vi "Configure Valve Output.vi"(8 "error in (no error)":errorcluster, 9 "valve output, %":sgl, 10 "node address (same)":u8, 11 "ProPar in":refnum<class "PL Bronkhorst ProPar.lvclass">) -> (0 "error out":errorcluster, 3 "ProPar out":refnum<class "PL Bronkhorst ProPar.lvclass">)   [LabVIEW 2015, in "PL Bronkhorst ProPar.lvclass"]
doc: "Configures valve output level of the specified <b>node</b>."
uses:
  PL Bronkhorst ProPar.lvclass
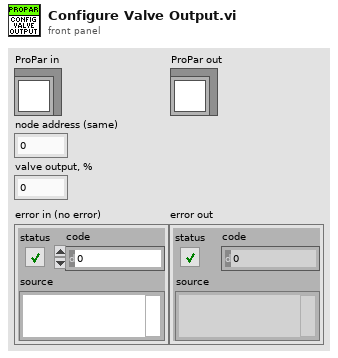
[diagram p1: front panel]
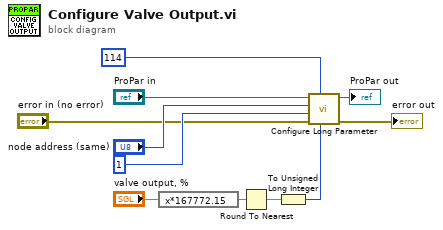
[diagram p0: block diagram]
diagram:
  n1 = expression code="x*167772.15"("valve output, %") -> (w10:sgl)
  n2 = Round To Nearest(number=w10) -> (nearest integer value=w9:sgl)
  n3 = To Unsigned Long Integer(number=w9) -> (unsigned 32bit integer=w2:u32)
  n4 = call "Configure Long Parameter.vi"("value"=w2, "process number"=u8 114, "error in (no error)"="error in (no error)", "parameter number"=u8 1 ("process number"), "node address (same)"="node address (same)", "ProPar in"="ProPar in") -> ("error out"=→"error out":errorcluster, "ProPar out"=→"ProPar out":refnum<class "PL Bronkhorst ProPar.lvclass">)  [unwired: 4 in]
